vi "Read Threshold.vi"(8 "error in (no error)":errorcluster, 11 "USAC Params in":refnum<class "USAC Params.lvclass">) -> (0 "error out":errorcluster, 2 "Threshold":dbl=1.5, 3 "USAC Params out":refnum<class "USAC Params.lvclass">)   [LabVIEW 2020, in "ar.lvlib" / "USAC Params.lvclass"]
uses:
  USAC Params.lvclass
  USAC Params.lvclass/USAC Params.ctl
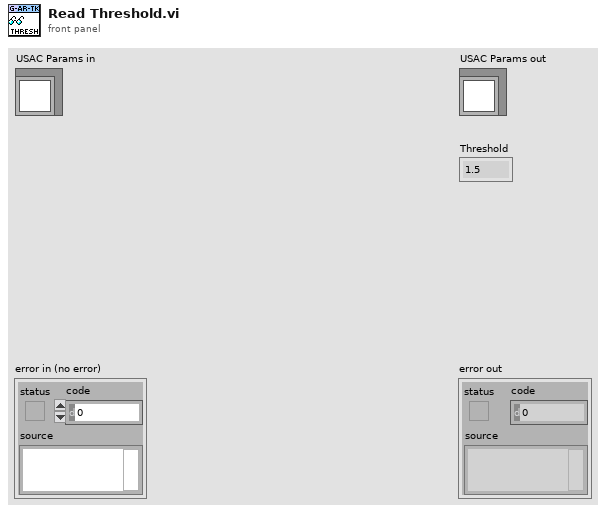
[diagram p1: front panel]
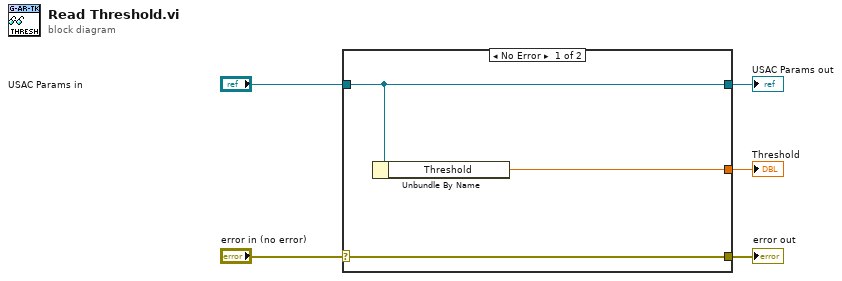
[diagram p0: block diagram]
diagram:
  n1 = case shown="No Error" "error in (no error)" {
    selector: "error in (no error)" -> [w8 w9]
    tunnel: [w8 w9] -> w4
    tunnel: [w7 w10] -> w2
    tunnel: "USAC Params in" -> [w7 w10]
    tunnel: [w6 _] -> w1
    frame No Error {
      n2 = Unbundle By Name(w7) -> ("Threshold"=w6:dbl)
    }
    frame Error {
    }
  }
  "error out" <- w4
  "USAC Params out" <- w2
  "Threshold" <- w1
